vi "Add Scale.vi"(8 "error in (no error)":errorcluster, 11 "Polynomial Scale configuration in":refnum<class "Polynomial Scale configuration.lvclass">) -> (0 "error out":errorcluster, 2 "new index":i32, 3 "Polynomial Scale configuration out":refnum<class "Polynomial Scale configuration.lvclass">)   [LabVIEW 2013, in "Polynomial Scale configuration.lvclass"]
uses:
  Polynomial Scale configuration.lvclass
  <vilib>/NI/DCAF Templates/DCAF Scaling/module/configuration/Scaling configuration.lvclass
  Polynomial Scale configuration.lvclass/Polynomial Scale configuration.ctl
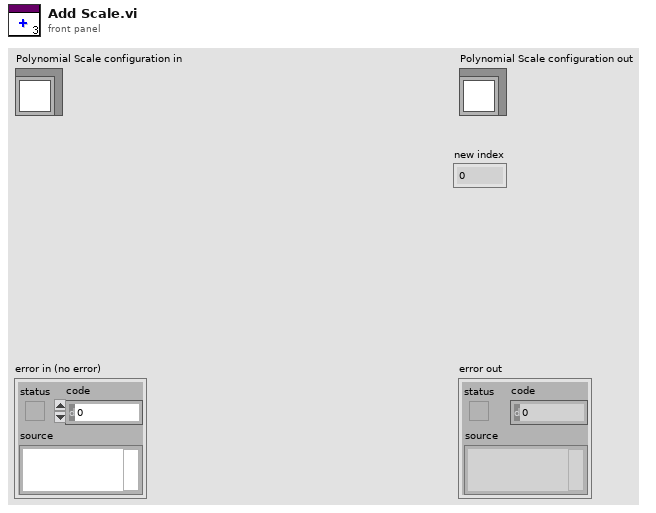
[diagram p1: front panel]
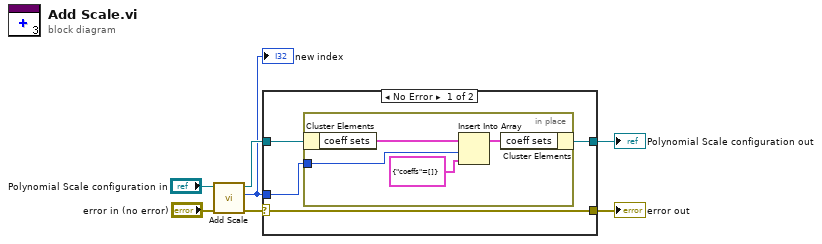
[diagram p0: block diagram]
diagram:
  n1 = call-parent "Add Scale.vi"("error in (no error)"="error in (no error)", "Scaling configuration in"="Polynomial Scale configuration in") -> ("error out"=w2:errorcluster, "new index"=w3:i32, "Scaling configuration out"=w5:refnum<class "Polynomial Scale configuration.lvclass">)  [unwired: 7 in]
  "new index" <- w3
  n2 = case shown="No Error" w2 {
    selector: w2 -> [w8 w16]
    tunnel: w5 -> [w11 w17]
    tunnel: [w10 w17] -> w4
    tunnel: w3 -> [w9 _]
    tunnel: [w8 w16] -> w1
    frame No Error {
      n3 = in-place {
        in-place-border: w9 -> [w13]
        n4 = in-place-cluster #1(w11) -> ("coeff sets"=w15:cluster{"coeffs":dbl[]}[])
        n5 = Insert Into Array(array=w15, index=w13, new element=cluster{"coeffs":dbl[]} {"coeffs"=[]} ("new element/subarray")) -> (w14:cluster{"coeffs":dbl[]}[])
        n6 = in-place-cluster #1("coeff sets"=w14) -> (w10:refnum<class "Polynomial Scale configuration.lvclass">)
      }
    }
    frame Error {
    }
  }
  "error out" <- w1
  "Polynomial Scale configuration out" <- w4
